vi "Remove Line From File.vi"(7 "Check Only? (f)":bool, 8 "Error In":errorcluster, 9 "Line":string="i2c-bcm2708", 10 "File Path":string="cat /etc/modules", 11 "Install LV Data":T1={"SSH Session"=refnum, "Status Log"="", "Detailed Log"="", "Credentials"={"Hostname or IP"="192.168.7.2", "Username"="root", "Password"=""}, "Target Info"={"OS Version"="", "CPU"="", "Systemd Version"="", "Internet Access"=FALSE, "Device Type"="", "LV Installed Ver"="", "LV Available Ver"="", "LV Upgrade Available"=FALSE, "Hostname"="", "NIC Info"=[]}, "Reboot Required?"=FALSE}) -> (0 "Error Out":errorcluster, 1 "Log":string, 2 "Line Previously Present?":bool, 3 "Install LV Data":T1={"SSH Session"=refnum, "Status Log"="", "Detailed Log"="", "Credentials"={"Hostname or IP"="192.168.7.2", "Username"="root", "Password"=""}, "Target Info"={"OS Version"="", "CPU"="", "Systemd Version"="", "Internet Access"=FALSE, "Device Type"="", "LV Installed Ver"="", "LV Available Ver"="", "LV Upgrade Available"=FALSE, "Hostname"="", "NIC Info"=[]}, "Reboot Required?"=FALSE})   [LabVIEW 2014, in "LMH-LINX.lvlib"]
uses:
  <vilib>/MakerHub/LINX/LMH-LINX.lvlib
  <vilib>/MakerHub/LINX/Private/Utilties/Target Management/Install LV Data.ctl
  C:/Program Files (x86)/National Instruments/LabVIEW 2014/vi.lib/MakerHub/LINX/Resources/Renci.SshNet.dll
  Resources/Renci.SshNet.dll
  <vilib>/MakerHub/LINX/Private/Utilties/Target Management/Target Info.ctl
  <vilib>/MakerHub/LINX/Private/Utilties/Target Management/NIC Info.ctl
  <vilib>/MakerHub/LINX/Private/Utilties/Target Management/NIC Mode.ctl
  <vilib>/regexp/Match Regular Expression.xnode
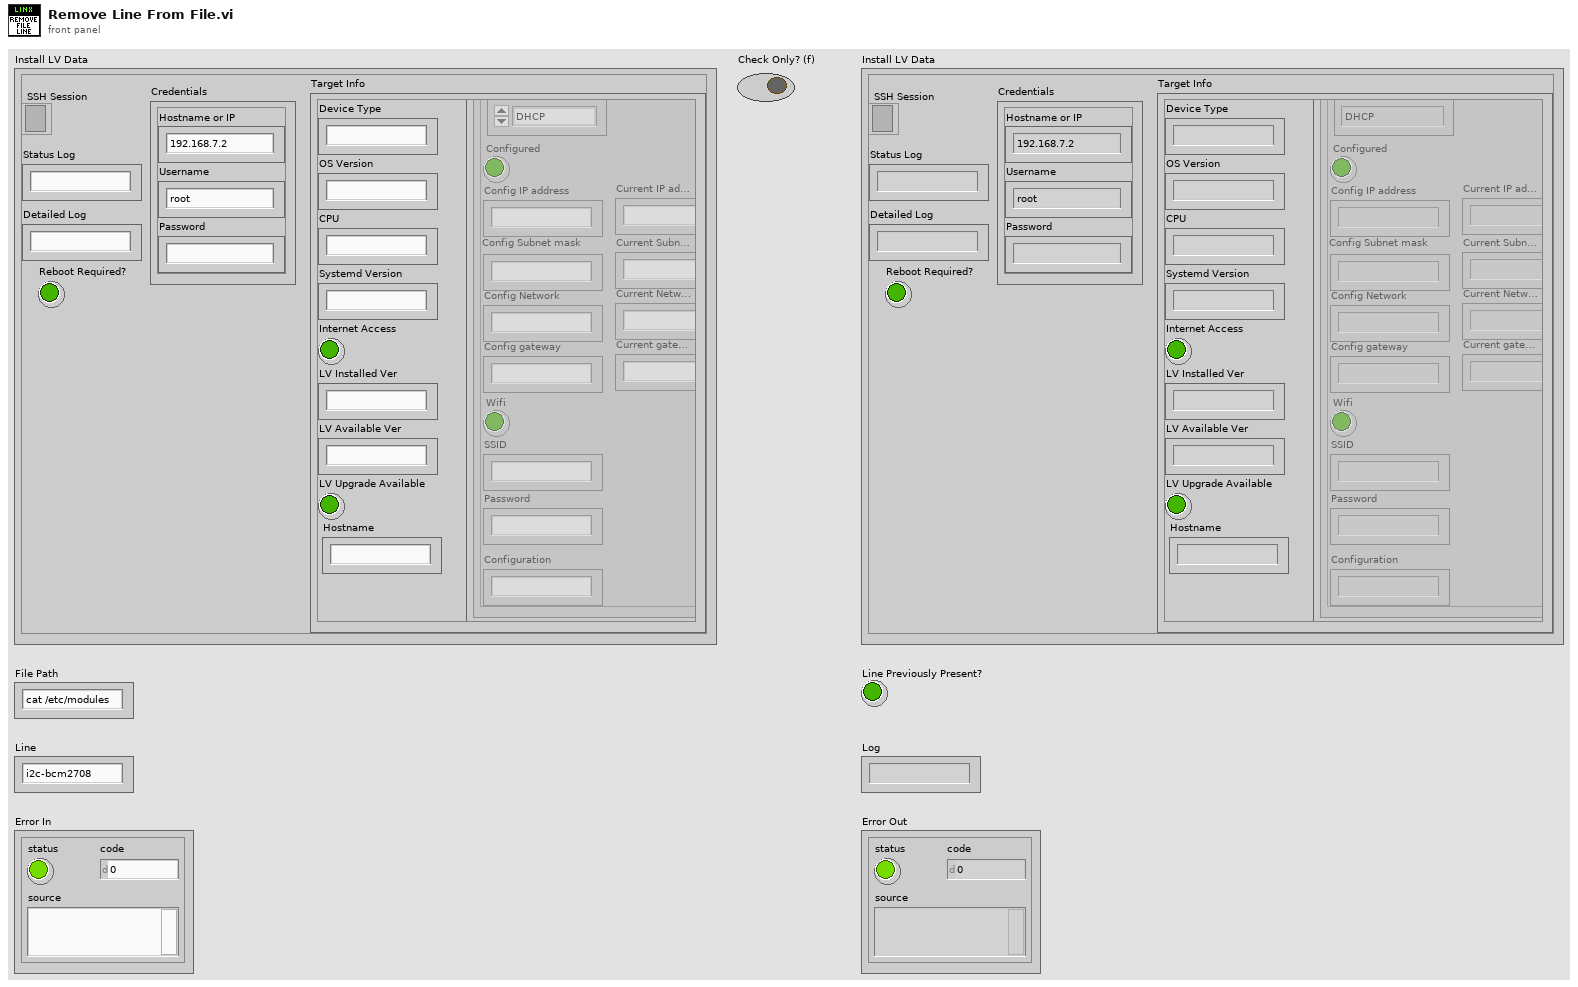
[diagram p1: front panel]
types:
  T1 = typedef "LMH-LINX.lvlib/Install LV Data.ctl" = cluster{"SSH Session":refnum<k24>, "Status Log":string, "Detailed Log":string, "Credentials":cluster{"Hostname or IP":string, "Username":string, "Password":string}, "Target Info":T2, "Reboot Required?":bool}
  T2 = typedef "LMH-LINX.lvlib/Target Info.ctl" = cluster{"OS Version":string, "CPU":string, "Systemd Version":string, "Internet Access":bool, "Device Type":string, "LV Installed Ver":string, "LV Available Ver":string, "LV Upgrade Available":bool, "Hostname":string, "NIC Info":T3[]}
  T3 = typedef "LMH-LINX.lvlib/NIC Info.ctl" = cluster{"Name":string, "NIC Mode":T4, "Configured":bool, "Config IP address":string, "Config Subnet mask":string, "Config Network":string, "Config gateway":string, "Wifi":bool, "SSID":string, "Password":string, "Configuration":string, "Current IP address":string, "Current Subnet mask":string, "Current gateway":string, "Current Network":string}
  T4 = typedef "LMH-LINX.lvlib/NIC Mode.ctl" = enum16{"DHCP", "Static", "Loopback"}
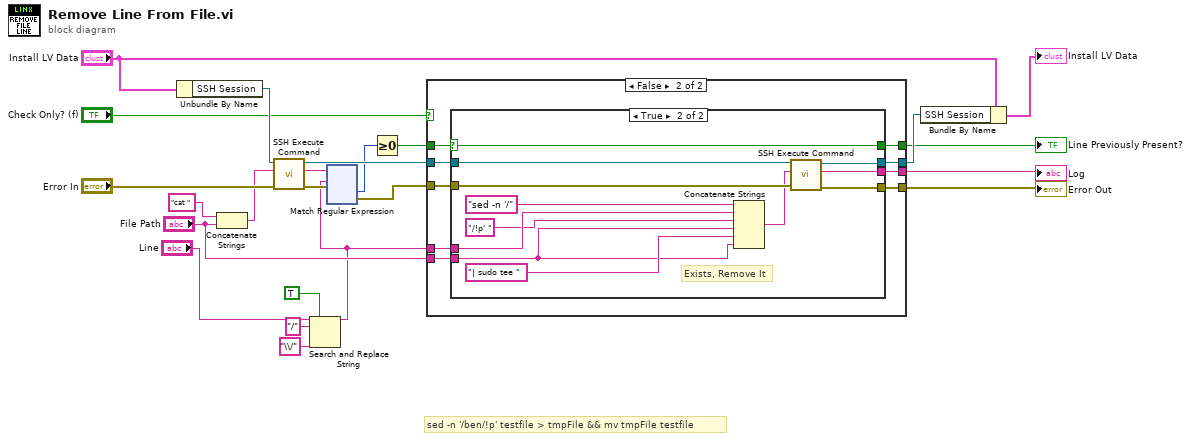
[diagram p0: block diagram]
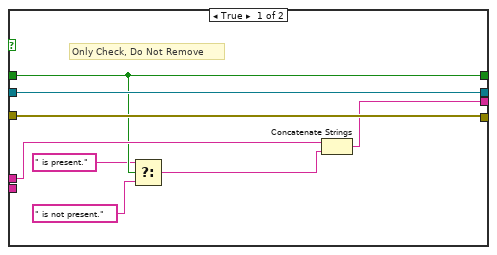
[diagram p2: hidden frame]
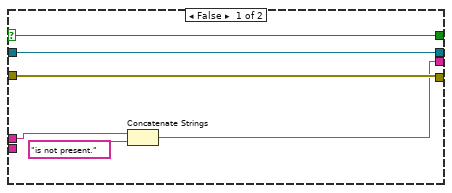
[diagram p3: hidden frame]
diagram:
  # "sed -n '/ben/!p' testfile > tmpFile && mv tmpFile testfile"
  n1 = Unbundle By Name("Install LV Data") -> ("SSH Session"=w21:refnum<k24>)
  n2 = Concatenate Strings("cat " ("string"), "File Path") -> (w12:string)
  n3 = call <vilib>:"SSH Execute Command.vi"("Error In"="Error In", "Command"=w12, "SSH Session"=w21) -> ("Error Out"=w18:errorcluster, "Std Out"=w14:string, "SSH Session"=w19:refnum<k24>)  [unwired: 6 in]
  n4 = Search and Replace String(replace all?=TRUE ("replace all? (F)"), input string="Line", search string="/", replace string="\\/" ("replace string (\"\")")) -> (result string=w1:string)  [unwired: 4 in, 3 out]
  n5 = xnode "Match Regular Expression"("input string"=w14, "regular expression"=w1, "error in"=w18) -> ("offset past match"=w16:i32, "error out"=w17:errorcluster)  [unwired: 3 in, 3 out]
  n6 = Greater Or Equal To 0?(x=w16) -> (x >= 0?=w15:bool)
  n7 = case shown="False" "Check Only? (f)" {
    tunnel: w19 -> [w31 w40]
    tunnel: w17 -> [w30 w39]
    tunnel: w15 -> [w27 w38]
    tunnel: w1 -> [w28 w37]
    tunnel: [w30 w36] -> w11
    tunnel: [w29 w35] -> w10
    tunnel: [w31 w34] -> w9
    tunnel: "File Path" -> [_ w33]
    tunnel: [w27 w32] -> w6
    frame True {
      # "Only Check, Do Not Remove"
      n8 = Select(t=" is present.", s=w27, f=" is not present.") -> (s? t:f=w24:string)
      n9 = Concatenate Strings(w28, w24) -> (w29:string)
    }
    frame False {
      n10 = case shown="True" w38 {
        selector: w38 -> [w44 w53]
        tunnel: [w41 w47] -> w35
        tunnel: [w46 w58] -> w36
        tunnel: [w45 w57] -> w34
        tunnel: w40 -> [w45 w56]
        tunnel: w39 -> [w46 w55]
        tunnel: w37 -> [w43 w51]
        tunnel: w33 -> [_ w48]
        tunnel: [w44 w53] -> w32
        frame False {
          n11 = Concatenate Strings(w43, "is not present." ("string")) -> (w41:string)
        }
        frame True {
          # "Exists, Remove It"
          n12 = Concatenate Strings("sed -n '/", w51, "/!p' ", w48, "| sudo tee ", w48) -> (w54:string)
          n13 = call <vilib>:"SSH Execute Command.vi"("Error In"=w55, "Command"=w54, "SSH Session"=w56) -> ("Error Out"=w58:errorcluster, "Std Out"=w47:string, "SSH Session"=w57:refnum<k24>)  [unwired: 6 in]
        }
      }
    }
  }
  "Log" <- w10
  "Error Out" <- w11
  "Line Previously Present?" <- w6
  n14 = Bundle By Name(cluster="Install LV Data", "SSH Session"=w9) -> (→"Install LV Data":T1)
